vi "save_ps.vi"(4 "Height":dbl, 6 "Rate":dbl, 7 "Comment":string, 8 "error in":errorcluster caption="error in (no error)", 11 "QPD Data":dbl[][](array[numeric])) -> (0 "error out":errorcluster)   [LabVIEW 2019]
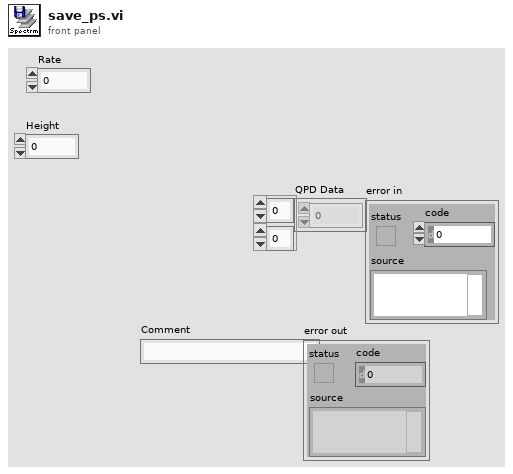
[diagram p1: front panel]
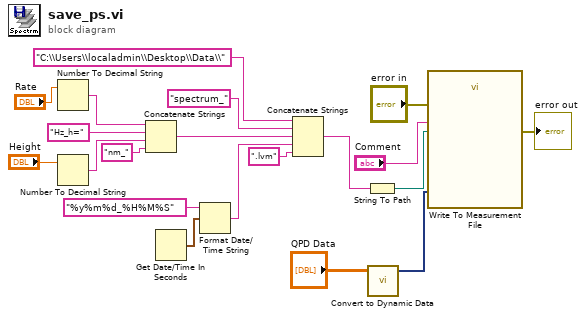
[diagram p0: block diagram]
diagram:
  n1 = Number To Decimal String(number="Rate") -> (decimal integer string=w3:string)  [unwired: 1 in]
  n2 = Number To Decimal String(number="Height") -> (decimal integer string=w1:string)  [unwired: 1 in]
  n3 = Concatenate Strings(w3, "Hz_h=" ("string"), w1, "nm_" ("string")) -> (w5:string)
  n4 = Get Date/Time In Seconds() -> (seconds since 1Jan1904=w17:timestamp)
  n5 = Format Date/Time String(time format string (%c)="%y%m%d_%H%M%S", seconds (now)=w17) -> (date/time string=w20:string)  [unwired: 1 in]
  n6 = Concatenate Strings("C:\\Users\\localadmin\\Desktop\\Data\\" ("string"), "spectrum_" ("string"), w5, w20, ".lvm" ("string")) -> (w19:string)
  n7 = String To Path(string=w19) -> (path=w16:path)
  n8 = call "Convert to Dynamic Data"("2D Array"="QPD Data") -> ("Dynamic Data Type"=w11:dynamicdata)  [unwired: 3 in]
  n9 = call "Write To Measurement File"("Signals"=w11, "error in (no error)"="error in", "Filename"=w16, "Comment"="Comment") -> ("error out"=→"error out":errorcluster)  [unwired: 13 in, 2 out]
